vi "Config Input Math.vi"(0 "VISA resource name":refnum<visa-resource-name>, 1 "Equation (0: y=mx+b)":u16(ring) items=["y=mx+b", "y=m(x+b)"], 2 "Input (0: A)":u16(ring) items=["A", "B", "C", "D"], 3 "Variable M Value (1.000)":dbl=1.0 min=-1000.0 max=1000.0 step=0.001 format="%.3f", 4 "Variable B Value (0.000)":dbl min=-100000000.0 max=100000000.0 step=0.001 format="%.3f", 5 "error in (no error)":errorcluster, 6 "Filter On/Off (F: Filter Off)":bool, 7 "X Source (0: Kelvin)":u16(ring) items=["Kelvin", "Celsius", "Sensor Units"], 10 "Points (2)":dbl=2.0 min=2.0 max=64.0 step=1.0, 11 "B Source (0: Varible B Value)":u16(ring) items=["Variable B Value", "+Setpoint 1", "-Setpoint 1", "+Setpoint 2", "-Setpoint 2"], 12 "Window (1)":dbl=1.0 min=1.0 max=10.0 step=1.0, 13 "Min/Max":T1 {"Source (0: Kelvin)" items=["Kelvin", "Celsius", "Sensor Units", "Linear Data"]; "On/Pause (0: On)" items=["On", "Pause"]}) -> (14 "VISA resource name out":refnum<visa-resource-name>, 19 "error out":errorcluster)   [LabVIEW 2019, in "Lake Shore Cryotronics 340.lvlib"]
doc: "This VI configures the math functions for the 340 inputs. Linear Equation, Min/Max, and Filter are all configured with this vi."
uses:
  Lake Shore Cryotronics 340.lvlib
panel:
  # "Linear Equation"
  # "Filter"
  # "Filter On\nFilter Off"
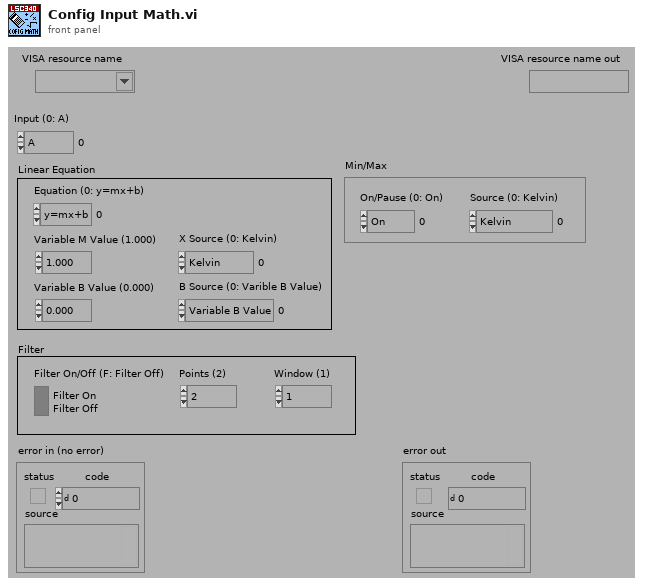
[diagram p1: front panel]
types:
  T1 = cluster{"On/Pause (0: On)":u16, "Source (0: Kelvin)":u16}
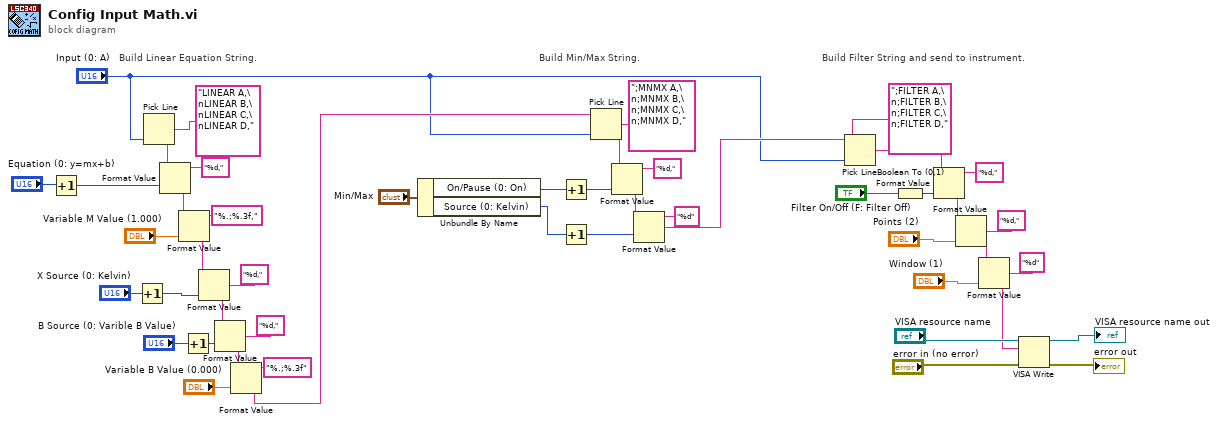
[diagram p0: block diagram]
diagram:
  # "Build Filter String and send to instrument."
  # "Build Min/Max String."
  # "Build Linear Equation String."
  n1 = Increment(x="Equation (0: y=mx+b)") -> (x+1=w32:u16)
  n2 = Increment(x="X Source (0: Kelvin)") -> (x+1=w43:u16)
  n3 = Pick Line(multi-line string="LINEAR A,\nLINEAR B,\nLINEAR C,\nLINEAR D,", line index="Input (0: A)") -> (output string=w33:string)  [unwired: 1 in]
  n4 = Format Value(string ("")=w33, format string="%d,", value (0)=w32) -> (output string=w36:string)
  n5 = Format Value(string ("")=w36, format string="%.;%.3f,", value (0)="Variable M Value (1.000)") -> (output string=w44:string)
  n6 = Increment(x="B Source (0: Varible B Value)") -> (x+1=w38:u16)
  n7 = Format Value(string ("")=w44, format string="%d,", value (0)=w43) -> (output string=w45:string)
  n8 = Format Value(string ("")=w45, format string="%d,", value (0)=w38) -> (output string=w48:string)
  n9 = Format Value(string ("")=w48, format string="%.;%.3f", value (0)="Variable B Value (0.000)") -> (output string=w22:string)
  n10 = Unbundle By Name("Min/Max") -> ("On/Pause (0: On)"=w2:u16, "Source (0: Kelvin)"=w1:u16)
  n11 = Increment(x=w2) -> (x+1=w29:u16)
  n12 = Increment(x=w1) -> (x+1=w28:u16)
  n13 = Pick Line(string ("")=w22, multi-line string=";MNMX A,\n;MNMX B,\n;MNMX C,\n;MNMX D,", line index="Input (0: A)") -> (output string=w25:string)
  n14 = Format Value(string ("")=w25, format string="%d,", value (0)=w29) -> (output string=w27:string)
  n15 = Format Value(string ("")=w27, format string="%d", value (0)=w28) -> (output string=w20:string)
  n16 = Pick Line(string ("")=w20, multi-line string=";FILTER A,\n;FILTER B,\n;FILTER C,\n;FILTER D,", line index="Input (0: A)") -> (output string=w16:string)
  n17 = Boolean To (0,1)(Boolean="Filter On/Off (F: Filter Off)") -> (0, 1=w17:i16)
  n18 = Format Value(string ("")=w16, format string="%d,", value (0)=w17) -> (output string=w15:string)
  n19 = Format Value(string ("")=w15, format string="%d,", value (0)="Points (2)") -> (output string=w10:string)
  n20 = Format Value(string ("")=w10, format string="%d", value (0)="Window (1)") -> (output string=w5:string)
  n21 = VISA Write(VISA resource name="VISA resource name", write buffer=w5, error in (no error)="error in (no error)") -> (VISA resource name out=→"VISA resource name out":refnum<visa-resource-name>, error out=→"error out":errorcluster)  [unwired: 1 out]
